vi "AIM664 Server Calls Test.vi"() -> ()   [LabVIEW 2020]
uses:
  src/AIM664LV.lvlib
panel:
  out "error out":errorcluster
  out "ResourceInfo":T1 {"PortMode" items=[" FDX_SINGLE", "FDX_REDUNDANT"]}
  in  "Input Cluster":T2={"SrvName"="local", "ResourceID"=1, "ResourceType"=0} {"ResourceType" items=["Board", "Port"]}
  in  "Input Cluster":T3={"SrvName"="local", "ClHostName"="local", "ClUser"="Brett", "ClApplication"="Test", "ClApplicationVersion"="V01.00", "ResourceID"=1, "Privileges"=4294967295} {"Privileges" items=["PRIVILEGES_ADMIN"=4294967295]}
  out "Output Cluster":T4
  in  "ServerRElement":u32=1
  out "NuOfResources":u32
  in  "SrvName":string="local"
  out "NuOfServers":u32
  # "ARINC 664 Server Check"
  # "Overview: Opens a reference to a server and login into the system.\nRequirement: One AIM ARINC-664 board with installed AIM ARINC 664 BSP.\nRestrictions: None.\nInstruction:\n1. Run the VI\n2. See results in the indicators"
  # "AXI FDX FdxInit Test"
  # "AiCountServerResources"
  # "GetServerResourcesCvi"
  # "QueryServerResourceCvi"
  # "FdxLoginCvi"
  # "FdxLogoutCvi"
  # "Input"
  # "Input"
  # "Input"
  # "Input"
  # "Input"
  # "Output"
  # "Output"
  # "Output"
  # "Output"
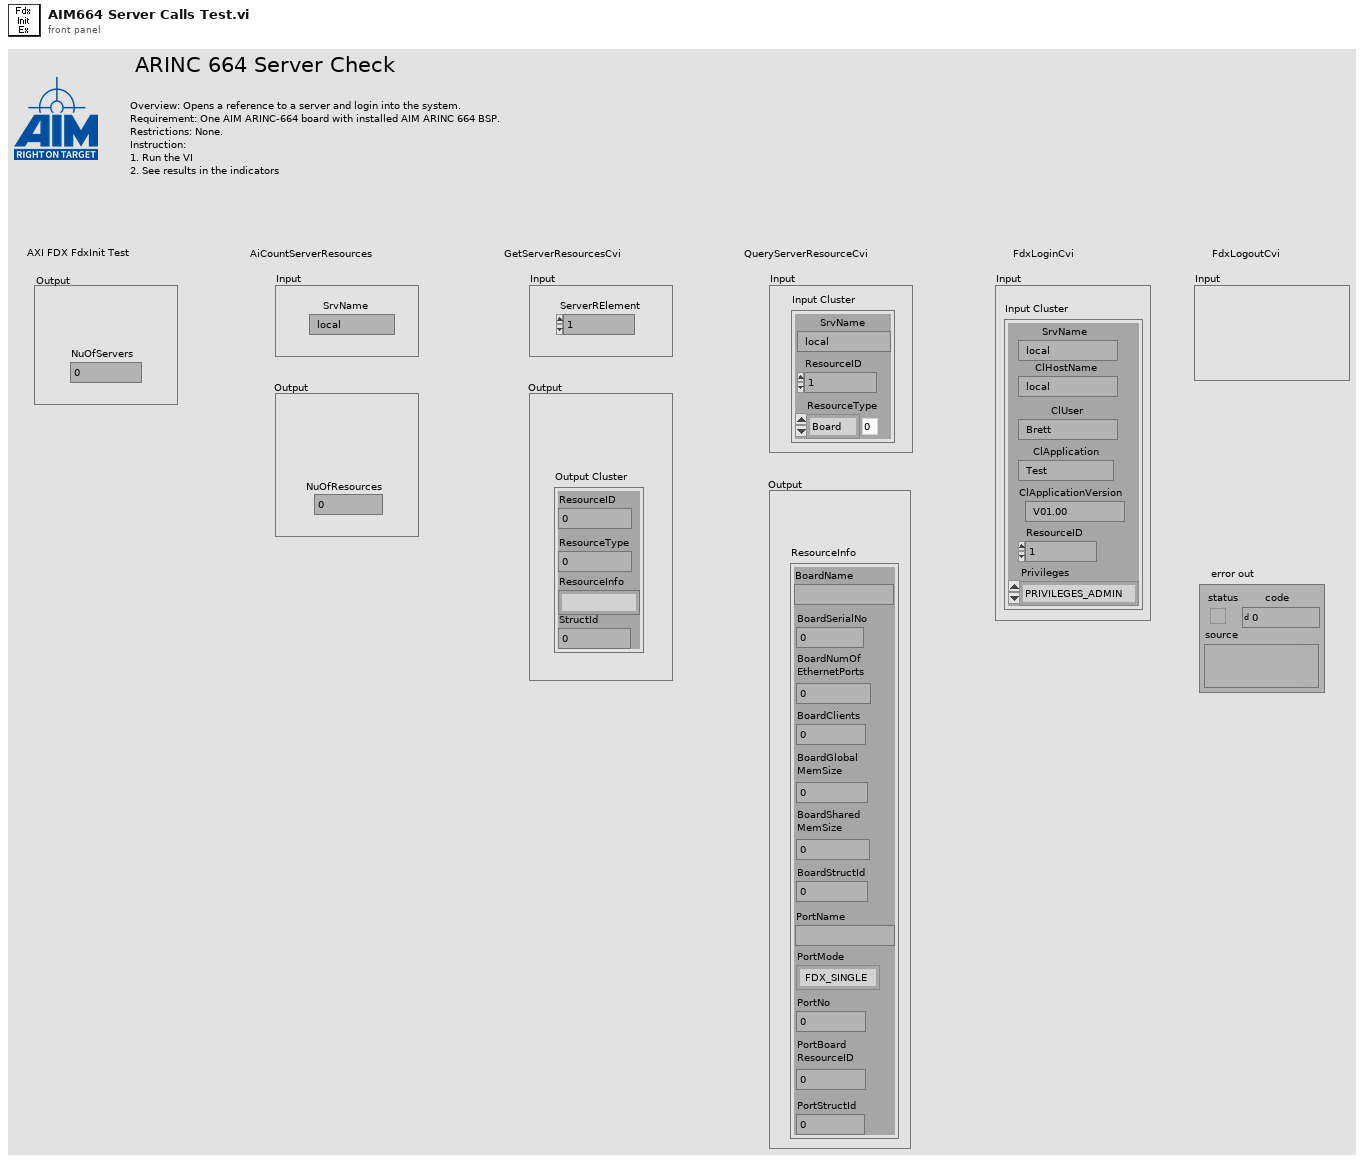
[diagram p1: front panel]
types:
  T1 = cluster{"BoardName":string, "BoardSerialNo":u32, "BoardNumOf\nEthernetPorts":u32, "BoardClients":u32, "BoardGlobal\nMemSize":u32, "BoardShared\nMemSize":u32, "BoardStructId":u32, "PortName":string, "PortMode":u32, "PortNo":u32, "PortBoard\nResourceID":u32, "PortStructId":u32}
  T2 = cluster{"SrvName":string, "ResourceID":u32, "ResourceType":u32}
  T3 = cluster{"SrvName":string, "ClHostName":string, "ClUser":string, "ClApplication":string, "ClApplicationVersion":string, "ResourceID":u32, "Privileges":u32}
  T4 = cluster{"ResourceID":u32, "ResourceType":u32, "ResourceInfo":string, "StructId":u32}
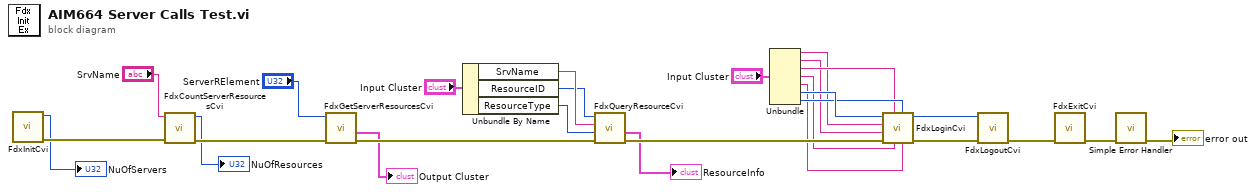
[diagram p0: block diagram]
diagram:
  n1 = call "FdxInitCvi.vi"() -> ("error out"=w27:errorcluster, "Number of Servers"=→"NuOfServers":u32)  [unwired: 10 in]
  n2 = call "FdxCountServerResourcesCvi.vi"("error in"=w27, "SrvName (local)"="SrvName") -> ("error out"=w26:errorcluster, "Number of Resources"=→"NuOfResources":u32)  [unwired: 8 in]
  n3 = call "FdxGetServerResourcesCvi.vi"("error in"=w26, "ServerRElement"="ServerRElement") -> ("error out"=w25:errorcluster, "ServerResourceInfo"=→"Output Cluster":T4)  [unwired: 4 in, 4 out]
  n4 = Unbundle By Name("Input Cluster") -> ("SrvName"=w13:string, "ResourceID"=w12:u32, "ResourceType"=w11:u32)
  n5 = call "FdxQueryResourceCvi.vi"("error in"=w25, "ResourceType"=w11, "SrvName"=w13, "ResourceID"=w12) -> ("error out"=w24:errorcluster, "ResourceInfo"=→"ResourceInfo":T1)  [unwired: 5 in, 1 out]
  n6 = Unbundle("Input Cluster") -> ("SrvName"=w6:string, "ClHostName"=w5:string, "ClUser"=w7:string, "ClApplication"=w4:string, "ClApplicationVersion"=w3:string, "ResourceID"=w9:u32, "Privileges"=w8:u32)
  n7 = call "FdxLoginCvi.vi"("ClApplicationVersion"=w3, "Privileges"=w8, "ClApplication"=w4, "ClUser"=w7, "error in"=w24, "ClHostName"=w5, "SrvName"=w6, "ResourceID"=w9) -> ("error out"=w23:errorcluster, "InstrumentHandle"=w20:u32)  [unwired: 2 in]
  n8 = call "FdxLogoutCvi.vi"("error in"=w23, "InstrumentHandle"=w20) -> ("error out"=w22:errorcluster)  [unwired: 9 in]
  n9 = call "FdxExitCvi.vi"("error in"=w22) -> ("error out"=w2:errorcluster)  [unwired: 10 in]
  n10 = call <vilib>:"Simple Error Handler.vi"("error in (no error)"=w2) -> ("error out"=→"error out":errorcluster)  [unwired: 4 in, 4 out]
